vi "Set-Image-offset-y.vi"(8 "error in (no error)":errorcluster, 9 "Offset Y in":i32, 10 "Image height":i32, 11 "PF_MV1-D1312-240 in":refnum<class "PF_MV1-D1312-240.lvclass">) -> (0 "error out":errorcluster, 1 "Offset Y":i32, 3 "PF_MV1-D1312-240 out":refnum<class "PF_MV1-D1312-240.lvclass">)   [LabVIEW 2013, in "CameraVision.lvlib" / "PF_MV1-D1312-240.lvclass"]
uses:
  PF_MV1-D1312-240.lvclass
  Camera.lvclass/Camera.ctl
  Read IMAQ Session.vi
  <userlib>/Photonfocus Toolkit/_Public/SubVIs/pf_Set_Camera_Property_Int.vi
  <userlib>/Photonfocus Toolkit/Photonfocus_Toolkit.lvlib
  Camera.lvclass
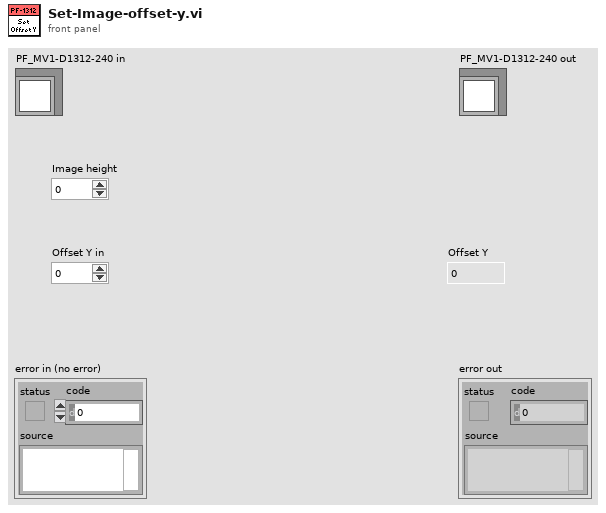
[diagram p1: front panel]
types:
  T1 = cluster{"Max. offset X":i32, "Max. offset Y":i32, "Offset step size X":i32, "Offset step size Y":i32}
  T2 = cluster{"Max. width":i32, "Max. height":i32, "Step size width":dbl, "Min. width":i32, "Min. height":i32, "Step size height":dbl}
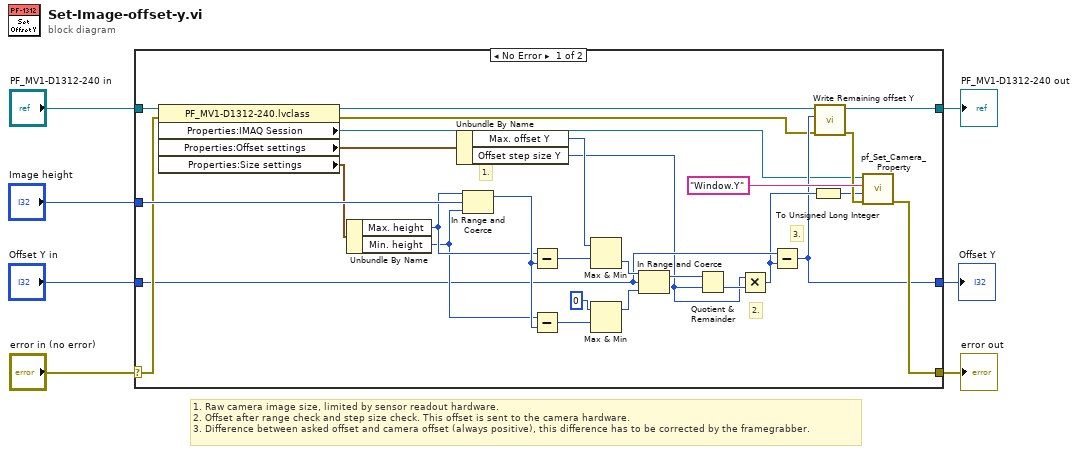
[diagram p0: block diagram]
diagram:
  # "1. Raw camera image size, limited by sensor readout hardware.\n2. Offset after range check and step size check. This offset is sent to the camera hardware.\n3. Difference between asked offset and camera offset (always positive), this difference has to be corrected by the framegrabber."
  n1 = case shown="No Error" "error in (no error)" {
    selector: "error in (no error)" -> [w23 w37]
    tunnel: [w34 w37] -> w6
    tunnel: [w18 w36] -> w4
    tunnel: "PF_MV1-D1312-240 in" -> [w35 w36]
    tunnel: "Image height" -> [w32 _]
    tunnel: [w14 _] -> w2
    tunnel: "Offset Y in" -> [w16 _]
    frame No Error {
      # "3."
      # "2."
      # "1."
      n2 = property class="PF_MV1-D1312-240.lvclass"(reference=w35, error in=w23) -> (reference out=w11:refnum<class "PF_MV1-D1312-240.lvclass">, error out=w12:errorcluster, "Properties:IMAQ Session"=w10:refnum<k11>, "Properties:Offset settings"=w13:T1, "Properties:Size settings"=w22:T2)
      n3 = Unbundle By Name(w22) -> ("Max. height"=w21:i32, "Min. height"=w20:i32)
      n4 = Unbundle By Name(w13) -> ("Max. offset Y"=w19:i32, "Offset step size Y"=w8:i32)
      n5 = In Range and Coerce(upper limit=w21, x=w32, lower limit=w20) -> (coerced(x)=w24:i32)  [unwired: 1 out]
      n6 = Subtract(x=w21, y=w24) -> (x-y=w31:i32)
      n7 = Subtract(x=w20, y=w24) -> (x-y=w29:i32)
      n8 = Max & Min(x=w19, y=w31) -> (min(x,y)=w30:i32)  [unwired: 1 out]
      n9 = Max & Min(x=0, y=w29) -> (max(x,y)=w27:i32)  [unwired: 1 out]
      n10 = In Range and Coerce(upper limit=w30, x=w16, lower limit=w27) -> (coerced(x)=w25:i32)  [unwired: 1 out]
      n11 = Quotient & Remainder(x=w25, y=w8) -> (floor(x/y)=w26:i32)  [unwired: 1 out]
      n12 = Multiply(x=w8, y=w26) -> (x*y=w15:i32)
      n13 = Subtract(x=w16, y=w15) -> (x-y=w14:i32)
      n14 = To Unsigned Long Integer(number=w15) -> (unsigned 32bit integer=w9:u32)
      n15 = call "Write Remaining offset Y.vi"("error in (no error)"=w12, "Offset Y"=w14, "Camera in"=w11) -> ("error out"=w17:errorcluster, "Camera out"=w18:refnum<class "PF_MV1-D1312-240.lvclass">)  [unwired: 7 in]
      n16 = call-poly <userlib>:"pf_Set_Camera_Property.vi"("error in (no error)"=w17, "Property Value"=w9, "Property Name"="Window.Y", "IMAQ Session in"=w10) -> ("error out"=w34:errorcluster)  [unwired: 5 in, 2 out]
    }
    frame Error {
    }
  }
  "error out" <- w6
  "PF_MV1-D1312-240 out" <- w4
  "Offset Y" <- w2
